vi "SetValue.vi"(9 "Edit Tree Items:Add Item":string, 10 "error in (no error)":errorcluster, 11 "TreeControl in":refnum<vi>) -> (2 "error out":errorcluster)   [LabVIEW 2021, in "Tree.lvlib" / "Tree.lvclass"]
uses:
  Tree.lvclass
  Tree.lvclass/Tree.ctl
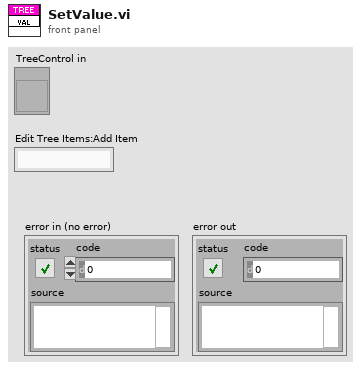
[diagram p1: front panel]
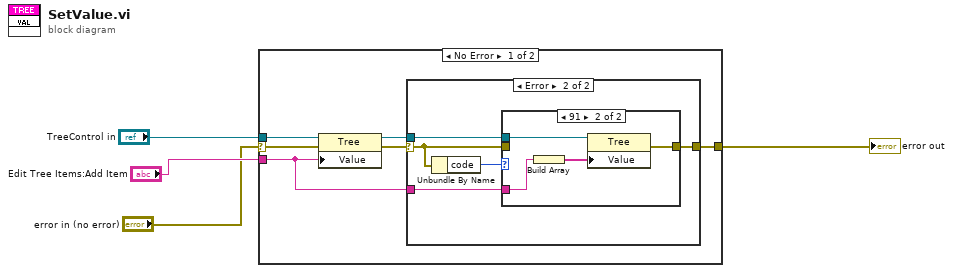
[diagram p0: block diagram]
diagram:
  n1 = case shown="No Error" "error in (no error)" {
    selector: "error in (no error)" -> [w8 w22]
    tunnel: [w7 w22] -> w4
    tunnel: "Edit Tree Items:Add Item" -> [w5 _]
    tunnel: "TreeControl in" -> [w10 _]
    frame No Error {
      n2 = property class="Tree"(reference=w10, error in=w8, "Value"=w5) -> (reference out=w9:refnum<vi>, error out=w6:errorcluster)
      n3 = case shown="Error" w6 {
        selector: w6 -> [w11 w13]
        tunnel: w9 -> [_ w16]
        tunnel: [w11 w14] -> w7
        tunnel: w5 -> [_ w12]
        frame No Error {
        }
        frame Error {
          n4 = Unbundle By Name(w13) -> ("code"=w15:i32)
          n5 = case shown="91" w15 {
            tunnel: w16 -> [_ w21]
            tunnel: [w17 w20] -> w14
            tunnel: w13 -> [w17 _]
            tunnel: w12 -> [_ w19]
            frame 0, Default {
            }
            frame 91 {
              n6 = Build Array(w19) -> (w18:string[])
              n7 = property class="Tree"(reference=w21, "Value"=w18) -> (error out=w20:errorcluster)  [unwired: 1 in, 1 out]
            }
          }
        }
      }
    }
    frame Error {
    }
  }
  "error out" <- w4
